vi "GPS Simple Navigate.vi"() -> ()   [LabVIEW 2009]
panel:
  out "Target Bearing":dbl
  in  "stop":bool
  in  "Current Latitude":dbl
  in  "Current Longitude":dbl
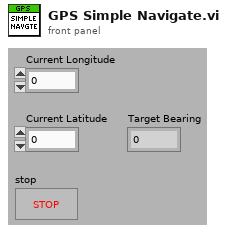
[diagram p1: front panel]
types:
  T1 = cluster{"[0]":void, "[1]":void, "[2]":void, "[3]":void, "[4]":void, "[5]":void, "[6]":void, "[7]":void, "[8]":void}
  T2 = cluster{"Current Latitude":dbl, "Current Longitude":dbl}
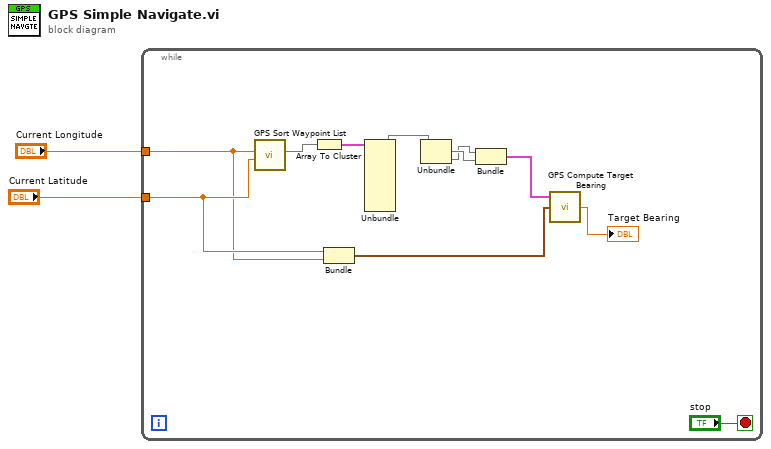
[diagram p0: block diagram]
diagram:
  n1 = while {
    tunnel: "Current Longitude" -> [w9]
    tunnel: "Current Latitude" -> [w10]
    stop <- "stop" stop-if-true
    n2 = call "GPS Sort Waypoint List.vi"(9:w10, "Current co-ordinate"=w9) -> (2:w13)  [unwired: 8 in, 1 out]
    n3 = Array To Cluster(array=w13) -> (cluster=w12:T1)
    n4 = Bundle("Current Latitude"=w10, "Current Longitude"=w9) -> (w5:T2)  [unwired: 1 in]
    n5 = Unbundle(w12) -> ("[0]"=w11)  [unwired: 8 out]
    n6 = Unbundle(w11) -> (w8, w7)  [unwired: 1 out]
    n7 = Bundle(w7, w8) -> (w4:cluster{void, void})  [unwired: 1 in]
    n8 = call "GPS Compute Target Bearing.vi"("Current Coordinates (Lat/Long)"=w5, "Target Coordinates (Lat/Long)"=w4) -> ("Target Bearing (degrees)"=→"Target Bearing":dbl)  [unwired: 3 in]
  }
